vi "ParseCommand2.vi"(0 "Command string":string) -> (1 "Command":string, 2 "Parameters":string[](array[string]))   [LabVIEW 2015]
uses:
  <vilib>/regexp/Match Regular Expression.xnode
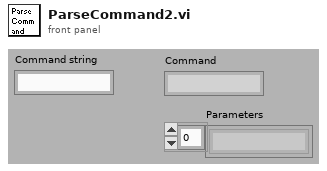
[diagram p1: front panel]
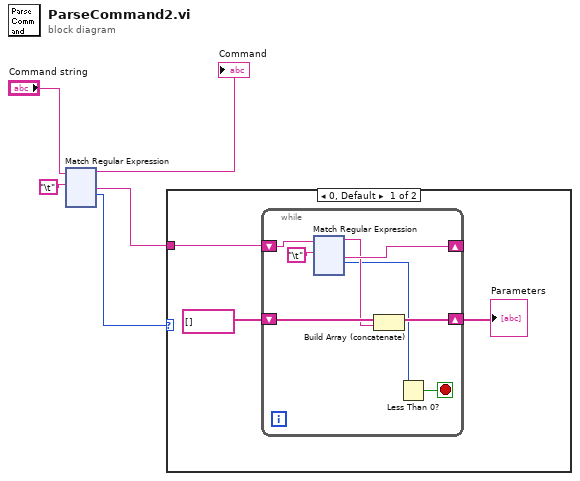
[diagram p0: block diagram]
diagram:
  n1 = xnode "Match Regular Expression"("input string"="Command string", "regular expression"="\t") -> ("before match"=→"Command":string, "after match"=w3:string, "offset past match"=w1:i32)  [unwired: 4 in, 2 out]
  n2 = case shown="0, Default" w1 {
    tunnel: w3 -> [w7 _]
    frame 0, Default {
      n3 = while {
        shift-right: [w14] -> _
        shift-left: w7 -> [w10]
        shift-right: [w11] -> w6
        shift-left: string[] [] -> [w13]
        stop <- w15 stop-if-true
        n4 = xnode "Match Regular Expression"("input string"=w10, "regular expression"="\t") -> ("before match"=w12:string, "after match"=w14:string, "offset past match"=w9:i32)  [unwired: 4 in, 2 out]
        n5 = Build Array (concatenate)(w13, w12) -> (w11:string[])
        n6 = Less Than 0?(x=w9) -> (x < 0?=w15:bool)
      }
      "Parameters" <- w6
    }
    frame -1 {
    }
  }
